vi "sub_score.vi"(8 "error in (no error)":errorcluster, 11 "Array In":bool[][](array[boolean])) -> (0 "error out":errorcluster, 2 "next state":bool)   [LabVIEW 2018]
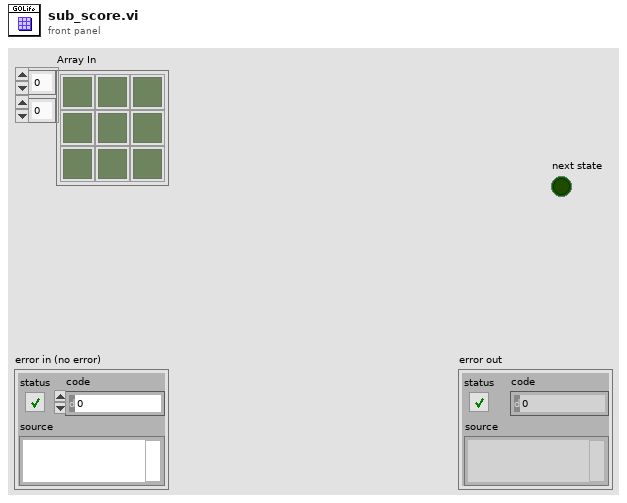
[diagram p1: front panel]
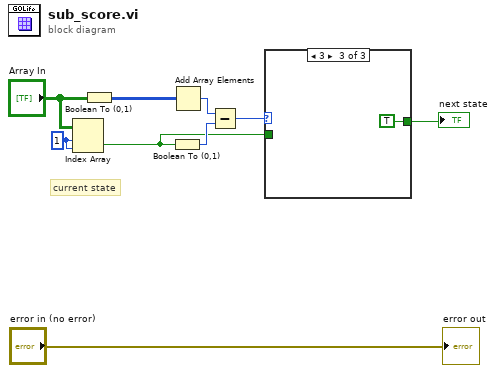
[diagram p0: block diagram]
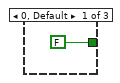
[diagram p2: hidden frame]
diagram:
  w8 = 1 ("index (row)")
  # "current state"
  n1 = Index Array(array="Array In", index (row)=w8, index (col)=w8) -> (element=w2:bool)
  n2 = Boolean To (0,1)(Boolean="Array In") -> (0, 1=w7:i16[][])
  n3 = Boolean To (0,1)(Boolean=w2) -> (0, 1=w5:i16)
  n4 = Add Array Elements(numeric array=w7) -> (sum=w6:i16)
  n5 = Subtract(x=w6, y=w5) -> (x-y=w4:i16)
  n6 = case shown="3" w4 {
    tunnel: [FALSE ("next state") w11 TRUE ("Boolean")] -> w3
    tunnel: w2 -> [_ w11 _]
    frame 0, Default {
    }
    frame 2 {
    }
    frame 3 {
    }
  }
  "next state" <- w3
  "error out" <- "error in (no error)"
